vi "motion.vi"(10 "location in":T1, 11 "location in":T1) -> (0 "upper white row position":i32, 1 "current peice column":i32, 2 "current peice row":i32, 3 "lower white column position":i32, 5 "allow [eice movement":bool)   [LabVIEW 2014]
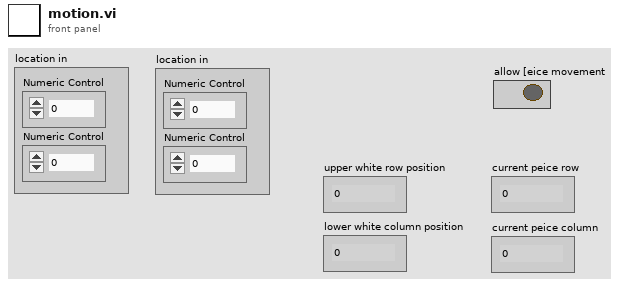
[diagram p1: front panel]
types:
  T1 = cluster{"Numeric Control":i32, "Numeric Control":i32}
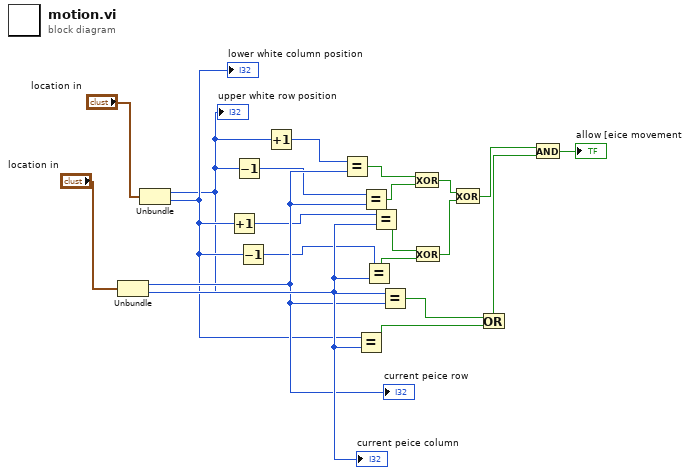
[diagram p0: block diagram]
diagram:
  n1 = Unbundle("location in") -> ("Numeric Control"=w15:i32, "Numeric Control"=w16:i32)
  "current peice column" <- w16
  "current peice row" <- w15
  n2 = Unbundle("location in") -> ("Numeric Control"=w13:i32, "Numeric Control"=w14:i32)
  "lower white column position" <- w14
  "upper white row position" <- w13
  n3 = Increment(x=w14) -> (x+1=w5:i32)
  n4 = Decrement(x=w13) -> (x-1=w4:i32)
  n5 = Decrement(x=w14) -> (x-1=w6:i32)
  n6 = Increment(x=w13) -> (x+1=w3:i32)
  n7 = Equal?(x=w3, y=w15) -> (x = y?=w7:bool)
  n8 = Equal?(x=w14, y=w16) -> (x = y?=w20:bool)
  n9 = Equal?(x=w4, y=w15) -> (x = y?=w8:bool)
  n10 = Equal?(x=w6, y=w16) -> (x = y?=w10:bool)
  n11 = Equal?(x=w5, y=w16) -> (x = y?=w9:bool)
  n12 = Equal?(x=w13, y=w15) -> (x = y?=w21:bool)
  n13 = Exclusive Or(1:w8, 2:w7) -> (0:w11:bool)
  n14 = Exclusive Or(1:w10, 2:w9) -> (0:w12:bool)
  n15 = Exclusive Or(1:w12, 2:w11) -> (0:w18:bool)
  n16 = Or(x=w21, y=w20) -> (x .or. y?=w19:bool)
  n17 = And(x=w18, y=w19) -> (x .and. y?=→"allow [eice movement":bool)
